vi "Save Image Module.vi"(8 "error in":errorcluster, 10 "Data":u64[](array[numeric]), 11 "Mode":T1) -> (0 "error out":errorcluster)   [LabVIEW 2013]
uses:
  Save Image Module Enum.ctl
  Debug/Debug Settings FG Enum.ctl
  Image Acquisition/Image Acquisition Settings FG Enum.ctl
  Image Processing/Mask ROI FG Enum.ctl
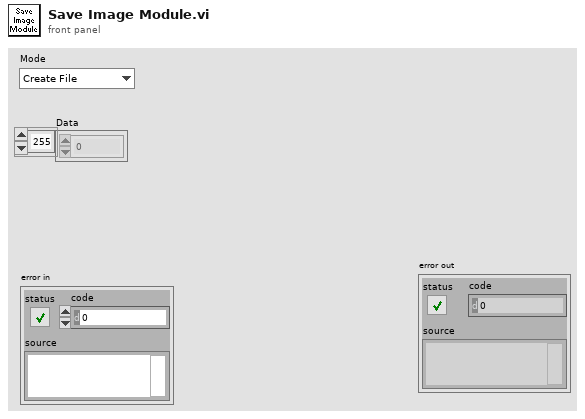
[diagram p1: front panel]
types:
  T1 = typedef "Save Image Module Enum.ctl" = enum16{"Create File", "Write to File", "Close File"}
  T2 = typedef "Debug Settings FG Enum.ctl" = enum16{"Read", "Write"}
  T3 = typedef "Debug Settings Cluster.ctl" = cluster{"Save Images?":bool, "Save Image Path":path}
  T4 = typedef "Mask ROI FG Enum.ctl" = enum16{"Read", "Write", "Enable Background", "Disable Background"}
  T5 = typedef "Image Acquisition Settings FG Enum.ctl" = enum16{"Read", "Write"}
  T6 = enum16{"open", "replace", "create", "open or create", "replace or create", "replace or create with confirmation"}
  T7 = typedef "Acquisition Settings Cluster.ctl" = cluster{"Image Width":u32, "Image Height":u32, "Frames To Acquire":u32, "Signal Mapping":enum8{"Standard", "Basler 10-tap", "Vosskühler 10-tap"}, "DMA Buffer Size\n(In Images)":u32}
  T8 = typedef "Mask ROI Cluster.ctl" = cluster{"left annulus":T9, "right annulus":T9, "Threshold Range":cluster{"Lower value":dbl, "Upper value":dbl}, "[Avg BG]":u8[], "Number of Sectors":u8, "Left ROI":T10, "Right ROI":T10, "Left Start Angle Duty Cycle":fxp<+,8,0>, "Left End Angle Duty Cycle":fxp<+,8,0>, "Right End Angle Duty Cycle":fxp<+,8,0>, "Right Start Angle Duty Cycle":fxp<+,8,0>, "[Sector ROIs]":T10[], "Consecutive Sector Threshold":u8}
  T9 = typedef "IMAQ Circle" = cluster{"Center X":i32, "Center Y":i32, "Inner Radius":i32, "Outer Radius":i32, "Start Angle":dbl, "End Angle":dbl}
  T10 = typedef "ROI Descriptor" = cluster{"Global Rectangle":i32[], "Contours":cluster{"ID":enum32{"External", "Internal"}, "Type":u32, "Coordinates":i32[]}[]}
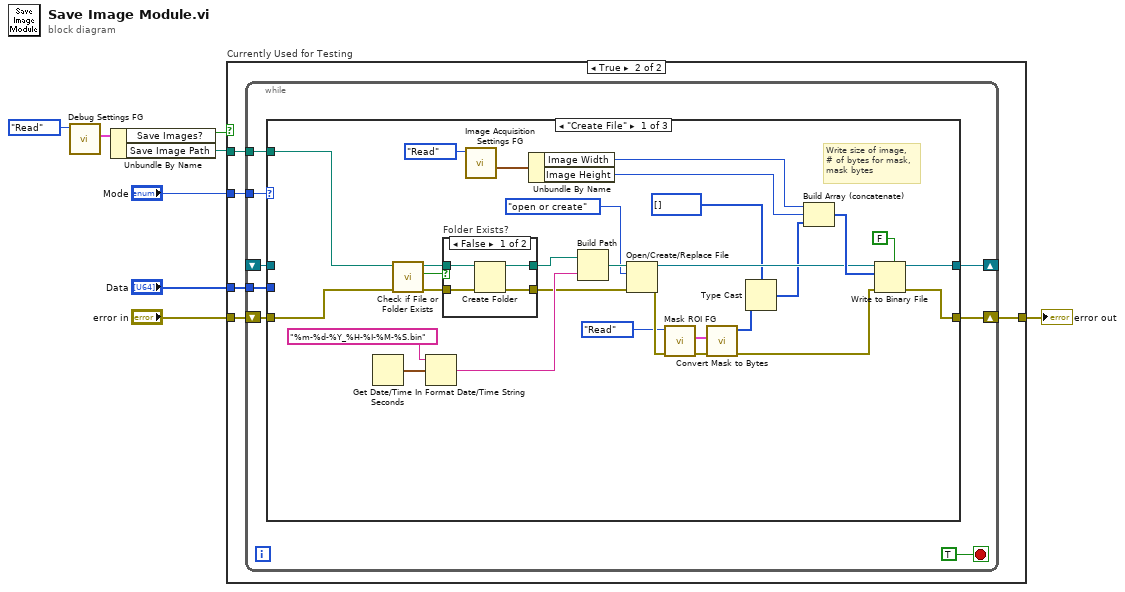
[diagram p0: block diagram]
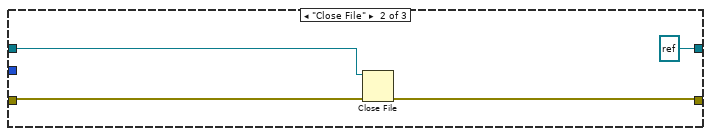
[diagram p4: hidden frame]
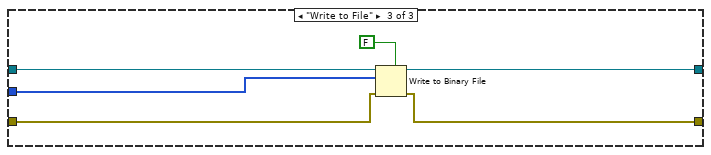
[diagram p5: hidden frame]
diagram:
  n1 = call "Debug Settings FG.vi"("Operation"=Debug_Settings_FG_Enum."Read") -> ("Debug Settings Out"=w4:T3)  [unwired: 9 in, 1 out]
  n2 = Unbundle By Name(w4) -> ("Save Images?"=w3:bool, "Save Image Path"=w1:path)
  n3 = case "Currently Used for Testing" shown="True" w3 {
    tunnel: "Mode" -> [_ w14]
    tunnel: "error in" -> [w9 w13]
    tunnel: [w9 w12] -> w6
    tunnel: "Data" -> [_ w11]
    tunnel: w1 -> [_ w10]
    frame False {
    }
    frame True {
      n4 = while {
        tunnel: w14 -> [w21]
        shift-right: [w18] -> w12
        shift-left: w13 -> [w20]
        shift-right: [w19] -> _
        shift-left: _ -> [w17]
        tunnel: w11 -> [w16]
        tunnel: w10 -> [w15]
        stop <- TRUE stop-if-true
        n5 = case shown="\"Create File\"" w21 {
          tunnel: w20 -> [w32 w61 w66]
          tunnel: [w35 refnum<file> refnum ("refnum out") w64] -> w19
          tunnel: [w34 w60 w65] -> w18
          tunnel: w17 -> [_ w59 w67]
          tunnel: w16 -> [_ _ w62]
          tunnel: w15 -> [w33 _ _]
          frame "Create File" {
            # "Write size of image,\n# of bytes for mask,\nmask bytes"
            n6 = Get Date/Time In Seconds() -> (seconds since 1Jan1904=w49:timestamp)
            n7 = call <vilib>:"Check if File or Folder Exists.vi"("error in (no error)"=w32, "path"=w33) -> ("error out"=w46:errorcluster, "file or folder exists?"=w48:bool, "dup path"=w47:path)  [unwired: 7 in]
            n8 = Format Date/Time String(time format string (%c)="%m-%d-%Y_%H-%I-%M-%S.bin", seconds (now)=w49) -> (date/time string=w51:string)  [unwired: 1 in]
            n9 = case "Folder Exists?" shown="False" w48 {
              tunnel: w47 -> [w55 w57]
              tunnel: w46 -> [w54 w56]
              tunnel: [w53 w56] -> w42
              tunnel: [w52 w57] -> w45
              frame False {
                n10 = Create Folder(path (use dialog)=w55, error in=w54) -> (created path=w52:path, error out=w53:errorcluster)  [unwired: 1 in, 1 out]
              }
              frame True {
              }
            }
            n11 = call "Image Acquisition Settings FG.vi"("Operation"=Image_Acquisition_Settings_FG_Enum."Read") -> ("Acquisition Settings Out"=w40:T7)  [unwired: 9 in, 1 out]
            n12 = Unbundle By Name(w40) -> ("Image Width"=w39:u32, "Image Height"=w38:u32)
            n13 = Build Path(base path=w45, name or relative path=w51) -> (appended path=w44:path)
            n14 = Open/Create/Replace File(file path (use dialog)=w44, error in=w42, operation (0:open)=T6."open or create") -> (refnum out=w30:refnum<file>, error out=w31:errorcluster)  [unwired: 3 in, 1 out]
            n15 = call "Mask ROI FG.vi"("error in (no error)"=w31, "Operation"=Mask_ROI_FG_Enum."Read") -> ("error out"=w28:errorcluster, "Mask ROI Out"=w27:T8)  [unwired: 8 in]
            n16 = call "Convert Mask to Bytes.vi"("error in (no error)"=w28, "Mask ROI In"=w27) -> ("error out"=w26:errorcluster, "Mask Bytes Out"=w24:u8[])  [unwired: 7 in, 1 out]
            n17 = Type Cast(type=u32[] [], x=w24) -> (*(type *) &x=w23:u32[])
            n18 = Build Array (concatenate)(w39, w38, w23) -> (w36:u32[])
            n19 = Write to Binary File(file (use dialog)=w30, data=w36, error in=w26, 5:FALSE ("prepend array or string size? (T)")) -> (refnum out=w35:refnum<file>, error out=w34:errorcluster)  [unwired: 2 in, 1 out]
          }
          frame "Close File" {
            n20 = Close File(refnum=w59, error in=w61) -> (error out=w60:errorcluster)  [unwired: 1 out]
          }
          frame "Write to File" {
            n21 = Write to Binary File(file (use dialog)=w67, data=w62, error in=w66, 5:FALSE ("prepend array or string size? (T)")) -> (refnum out=w64:refnum<file>, error out=w65:errorcluster)  [unwired: 2 in, 1 out]
          }
        }
      }
    }
  }
  "error out" <- w6
